vi "SetFrameRate.vi"(8 "error in (no error)":errorcluster, 10 "Frame Rate (hex code)":u8 format="%.0x", 11 "CameraSim in":refnum<class "CameraI2COUSB.lvclass">) -> (0 "error out":errorcluster, 3 "CameraSim out":refnum<class "CameraI2COUSB.lvclass">)   [LabVIEW 2020, in "Camera.lvlib" / "CameraI2COUSB.lvclass"]
uses:
  CameraI2COUSB.lvclass
  CameraI2COUSB.lvclass/CameraI2COUSB.ctl
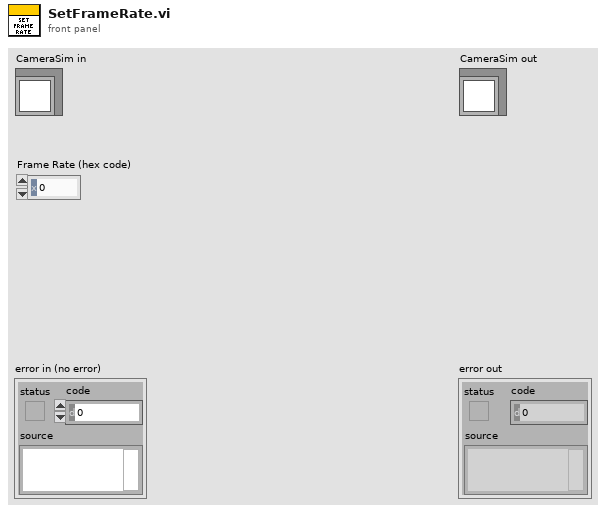
[diagram p1: front panel]
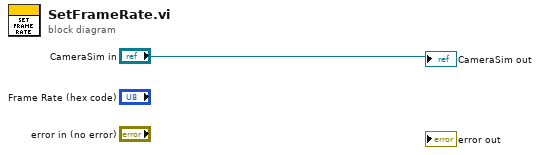
[diagram p0: block diagram]
diagram:
  "CameraSim out" <- "CameraSim in"
